vi "enableFIFO.vi"(0 "enable":bool) -> ()   [LabVIEW 2016]
uses:
  #defines.ctl
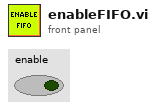
[diagram p1: front panel]
types:
  T1 = typedef "#defines.ctl" = i8
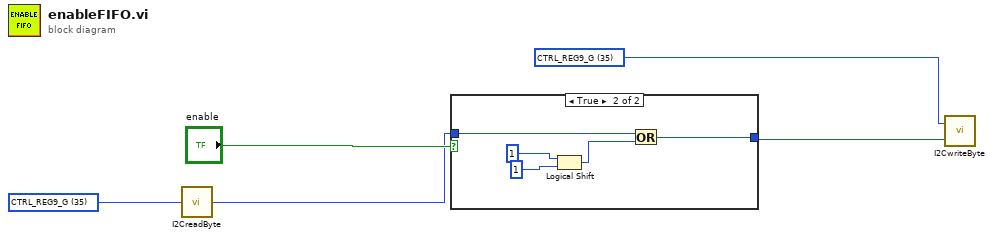
[diagram p0: block diagram]
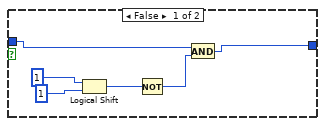
[diagram p2: hidden frame]
diagram:
  w1 = T1 35 items=["CTRL_REG9_G"=35, "STATUS_REG_1"=39, "OUT_X_L_XL"=40, "FIFO_CTRL"=46, "FIFO_SRC"=47, "CTRL_REG4_G"=30, "OUT_X_L_G"=24, "OUT_TEMP_L"=21, "INT_GEN_SRC_G"=20, "ORIENT_CFG_G"=19, "CTRL_REG3_G"=18, "CTRL_REG2_G"=17, "CTRL_REG1_G"=16, "WHO_AM_I_XG"=15] ("Ring")
  w3 = T1 35 items=["CTRL_REG9_G"=35, "STATUS_REG_1"=39, "OUT_X_L_XL"=40, "FIFO_CTRL"=46, "FIFO_SRC"=47, "CTRL_REG4_G"=30, "OUT_X_L_G"=24, "OUT_TEMP_L"=21, "INT_GEN_SRC_G"=20, "ORIENT_CFG_G"=19, "CTRL_REG3_G"=18, "CTRL_REG2_G"=17, "CTRL_REG1_G"=16, "WHO_AM_I_XG"=15] ("Ring")
  n1 = call "I2CreadByte.vi"("subAddress"=w3) -> ("data"=w4:u8)
  n2 = case shown="True" "enable" {
    tunnel: w4 -> [w11 w13]
    tunnel: [w6 w12] -> w2
    frame False {
      n3 = Logical Shift(y=i16 1, x=u32 1) -> (x << y=w8:u32)
      n4 = Not(x=w8) -> (.not. x?=w7:u32)
      n5 = And(x=w11, y=w7) -> (x .and. y?=w6:u32)
    }
    frame True {
      n6 = Logical Shift(y=i16 1, x=u32 1) -> (x << y=w14:u32)
      n7 = Or(x=w13, y=w14) -> (x .or. y?=w12:u32)
    }
  }
  n8 = call "I2CwriteByte.vi"("data"=w2, "subAddress"=w1) -> ()  [unwired: 1 in]
